vi "format_data.vi"(1 "data":string, 2 "name":string) -> (0 "concatenated string":string)   [LabVIEW 2013, in "TCP_IP.lvclass"]
uses:
  TCP_IP.lvclass
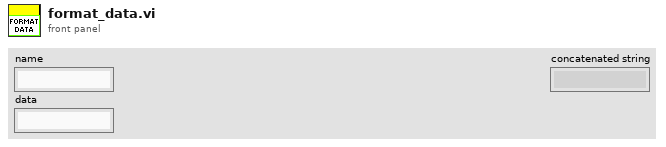
[diagram p1: front panel]
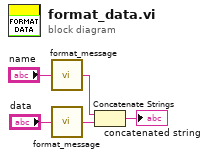
[diagram p0: block diagram]
diagram:
  n1 = call "format_message.vi"("messge"="name") -> ("concatenated string"=w3:string)
  n2 = call "format_message.vi"("messge"="data") -> ("concatenated string"=w2:string)
  n3 = Concatenate Strings(w3, w2) -> (→"concatenated string":string)
